vi "test_av_koeff.vi"(1 "s":bool, 2 "in":dbl[](array[numeric]), 4 "FIR Coefficients":dbl[](array[numeric])) -> (6 "out":dbl[](array[numeric]))   [LabVIEW 2015]
uses:
  <vilib>/Analysis/3filter.llb/FIR Filter (DBL).vi
  <vilib>/Analysis/NI_AALBase.lvlib
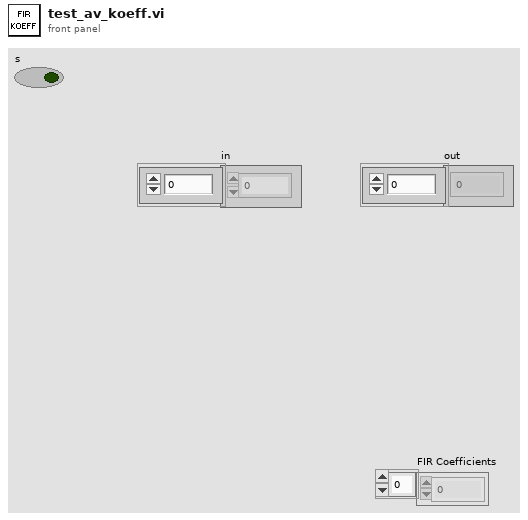
[diagram p1: front panel]
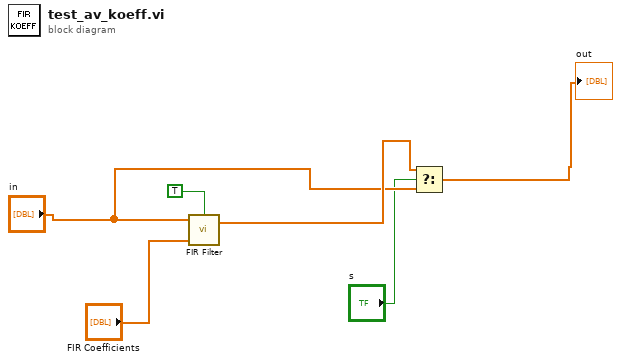
[diagram p0: block diagram]
diagram:
  n1 = call-poly <vilib>:"FIR Filter.vi"("init/cont (init:F)"=TRUE, "FIR Coefficients"="FIR Coefficients", "X"="in") -> ("Filtered X"=w3:dbl[])  [unwired: 1 in, 1 out]
  n2 = Select(t=w3, s="s", f="in") -> (s? t:f=→"out":dbl[])
